vi "_FPGA Auxiliary Update.vi"(5 "Setting Value":sgl, 6 "Command Type":i32) -> (0 "error out":errorcluster, 1 "Return Value":string)   [LabVIEW 2015]
uses:
  Type/_Syringe Pump Command.ctl
  Type/_Pump Parameter.ctl
  _RT Global.vi
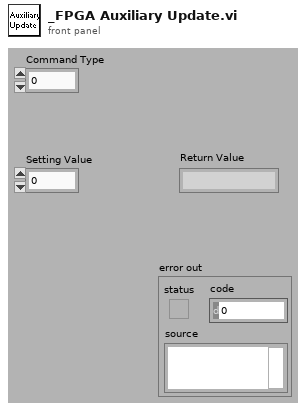
[diagram p1: front panel]
types:
  T1 = typedef "_Syringe Pump Command.ctl" = enum16{"start", "stop", "pause", "restart", "help", "set units", "set diameter", "set rate", "set time", "set volume", "set delay", "save setting", "read limit parameter", "view parameter", "status"}
  T2 = typedef "_Pump Parameter.ctl" = enum16{"Turn Pump Motor On", "Turn Pump Motor Off", "Read Pump Oil Deficiency", "Read Rotation Switch Point Attained", "Read Ele. Drive Over Temperature", "Read Pump Over Temperature", "Read Set Rotation Speed Attained", "Read Turbopump Accelerates", "Read Actual Rotation Speed in Hz", "Read Motor Current in A", "Read Operating Hours in h", "Read Motor Voltage in V", "Read Motor Power in W", "Set Rotation Speed Switchpoint in %", "Clear Error", "Read Error Code", "Read Bearing Temperature", "Read Hardware Version", "Read Firmware Version", "Read Operating Hours (Drive)", "Read Rotational Speed (rpm)", "Read Power Stage Temperature", "Read Electronics Temperature", "Read Upper Pump Temperature", "Read Motor Temperature", "Read Error Code History, 1", "Read Error Code History, 2", "Read Error Code History, 3", "Read Error Code History, 4", "Read Error Code History, 5", "Read Error Code History, 6", "Read Error Code History, 7", "Read Error Code History, 8", "Read Error Code History, 9", "Read Error Code History, 10"}
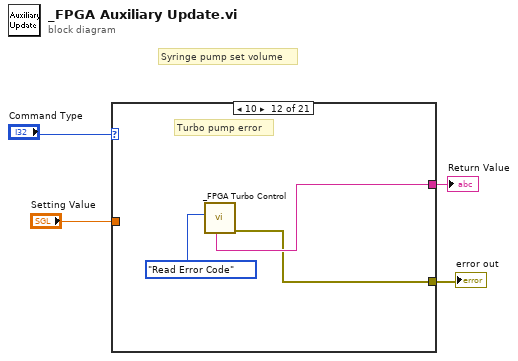
[diagram p0: block diagram]
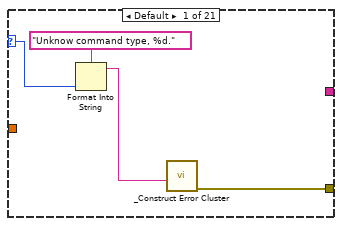
[diagram p2: hidden frame]
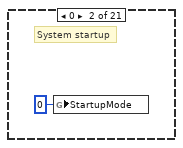
[diagram p3: hidden frame]
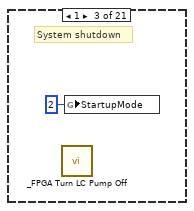
[diagram p4: hidden frame]
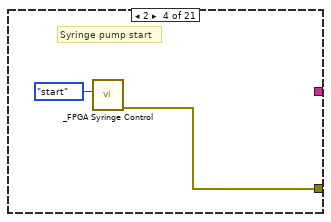
[diagram p5: hidden frame]
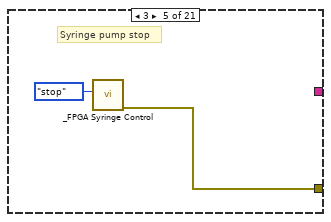
[diagram p6: hidden frame]
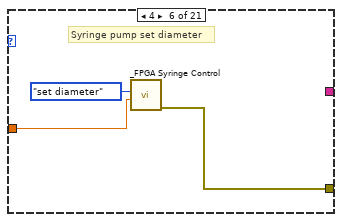
[diagram p7: hidden frame]
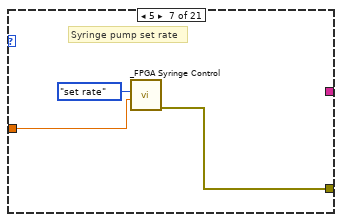
[diagram p8: hidden frame]
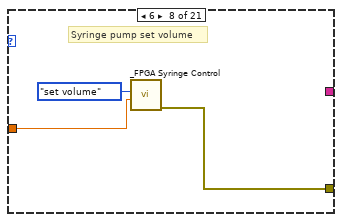
[diagram p9: hidden frame]
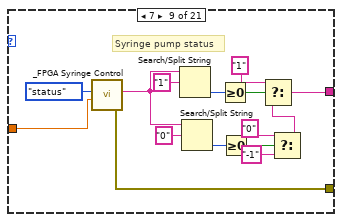
[diagram p10: hidden frame]
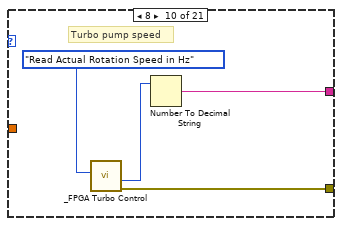
[diagram p11: hidden frame]
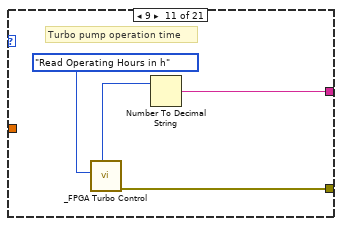
[diagram p12: hidden frame]
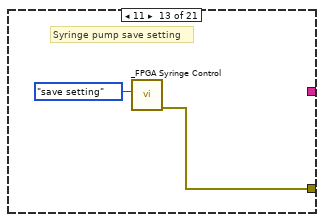
[diagram p13: hidden frame]
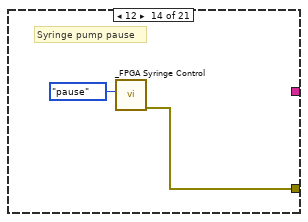
[diagram p14: hidden frame]
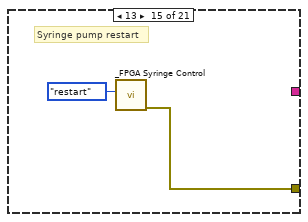
[diagram p15: hidden frame]
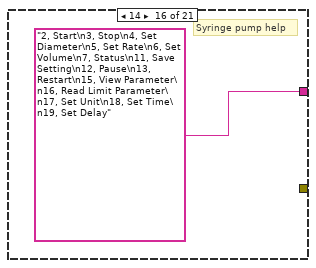
[diagram p16: hidden frame]
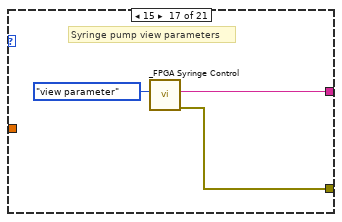
[diagram p17: hidden frame]
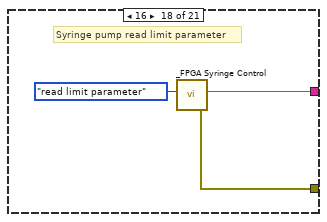
[diagram p18: hidden frame]
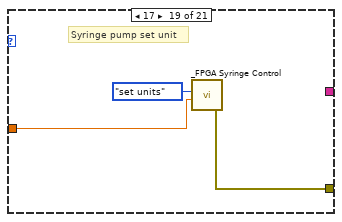
[diagram p19: hidden frame]
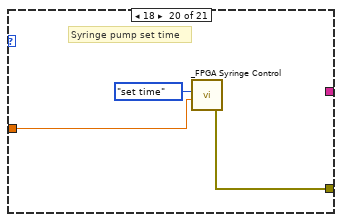
[diagram p20: hidden frame]
diagram:
  # "Syringe pump set volume"
  n1 = case shown="10" "Command Type" {
    selector: "Command Type" -> [w8 _ _ _ _ _ _ _ _ _ _ _ _ _ _ _ _ _ _ _ _]
    tunnel: [w5 _ _ w12 w14 w17 w20 w23 w38 w41 w45 w47 w51 w53 w55 _ w59 w62 w65 w68 w71] -> w2
    tunnel: "Setting Value" -> [_ _ _ _ _ w15 w18 w21 w36 _ _ _ _ _ _ _ _ _ w63 w66 w69]
    tunnel: [_ _ _ _ _ _ _ _ w25 w39 w44 w48 _ _ _ "2, Start\n3, Stop\n4, Set Diameter\n5, Set Rate\n6, Set Volume\n7, Status\n11, Save Setting\n12, Pause\n13, Restart\n15, View Parameter\n16, Read Limit Parameter\n17, Set Unit\n18, Set Time\n19, Set Delay" ("Reply") w57 w60 _ _ _] -> w1
    frame Default {
      n2 = Format Into String(format string="Unknow command type, %d.", w8) -> (resulting string=w6:string)  [unwired: 2 in, 1 out]
      n3 = call "_Construct Error Cluster.vi"("reason"=w6) -> ("error out"=w5:errorcluster)  [unwired: 3 in, 3 out]
    }
    frame 0 {
      # "System startup"
      n4 = global write "_RT Global.vi" "StartupMode"(u8 0 ("StartupMode")) -> ()
    }
    frame 1 {
      # "System shutdown"
      n5 = call "_FPGA Turn LC Pump Off.vi"() -> ()  [unwired: 2 in]
      n6 = global write "_RT Global.vi" "StartupMode"(u8 2 ("StartupMode")) -> ()
    }
    frame 2 {
      # "Syringe pump start"
      n7 = call "_FPGA Syringe Control.vi"("Pump Command"=_Syringe_Pump_Command."start") -> ("error out"=w12:errorcluster)  [unwired: 5 in, 2 out]
    }
    frame 3 {
      # "Syringe pump stop"
      n8 = call "_FPGA Syringe Control.vi"("Pump Command"=_Syringe_Pump_Command."stop") -> ("error out"=w14:errorcluster)  [unwired: 5 in, 2 out]
    }
    frame 4 {
      # "Syringe pump set diameter"
      n9 = call "_FPGA Syringe Control.vi"("Input Value"=w15, "Pump Command"=_Syringe_Pump_Command."set diameter") -> ("error out"=w17:errorcluster)  [unwired: 4 in, 2 out]
    }
    frame 5 {
      # "Syringe pump set rate"
      n10 = call "_FPGA Syringe Control.vi"("Input Value"=w18, "Pump Command"=_Syringe_Pump_Command."set rate") -> ("error out"=w20:errorcluster)  [unwired: 4 in, 2 out]
    }
    frame 6 {
      # "Syringe pump set volume"
      n11 = call "_FPGA Syringe Control.vi"("Input Value"=w21, "Pump Command"=_Syringe_Pump_Command."set volume") -> ("error out"=w23:errorcluster)  [unwired: 4 in, 2 out]
    }
    frame 7 {
      # "Syringe pump status"
      n12 = call "_FPGA Syringe Control.vi"("Input Value"=w36, "Pump Command"=_Syringe_Pump_Command."status") -> ("error out"=w38:errorcluster, "Reply"=w26:string)  [unwired: 4 in, 1 out]
      n13 = Search/Split String(string=w26, search string/char (-)="1") -> (offset of match=w33:i32)  [unwired: 3 out]
      n14 = Search/Split String(string=w26, search string/char (-)="0") -> (offset of match=w32:i32)  [unwired: 3 out]
      n15 = Greater Or Equal To 0?(x=w33) -> (x >= 0?=w31:bool)
      n16 = Greater Or Equal To 0?(x=w32) -> (x >= 0?=w29:bool)
      n17 = Select(t="0" ("search string/char (-)"), s=w29, f="-1") -> (s? t:f=w24:string)
      n18 = Select(t="1" ("search string/char (-)"), s=w31, f=w24) -> (s? t:f=w25:string)
    }
    frame 8 {
      # "Turbo pump speed"
      n19 = call "_FPGA Turbo Control.vi"("Command"=_Pump_Parameter."Read Actual Rotation Speed in Hz") -> ("error out"=w41:errorcluster, "Speed"=w40:i32)  [unwired: 3 in, 4 out]
      n20 = Number To Decimal String(number=w40) -> (decimal integer string=w39:string)  [unwired: 1 out]
    }
    frame 9 {
      # "Turbo pump operation time"
      n21 = call "_FPGA Turbo Control.vi"("Command"=_Pump_Parameter."Read Operating Hours in h") -> ("error out"=w45:errorcluster, "Time"=w43:i32)  [unwired: 3 in, 4 out]
      n22 = Number To Decimal String(number=w43) -> (decimal integer string=w44:string)  [unwired: 1 out]
    }
    frame 10 {
      # "Turbo pump error"
      n23 = call "_FPGA Turbo Control.vi"("Command"=_Pump_Parameter."Read Error Code") -> ("error out"=w47:errorcluster, "Error Code"=w48:string)  [unwired: 3 in, 4 out]
    }
    frame 11 {
      # "Syringe pump save setting"
      n24 = call "_FPGA Syringe Control.vi"("Pump Command"=_Syringe_Pump_Command."save setting") -> ("error out"=w51:errorcluster)  [unwired: 5 in, 2 out]
    }
    frame 12 {
      # "Syringe pump pause"
      n25 = call "_FPGA Syringe Control.vi"("Pump Command"=_Syringe_Pump_Command."pause") -> ("error out"=w53:errorcluster)  [unwired: 5 in, 2 out]
    }
    frame 13 {
      # "Syringe pump restart"
      n26 = call "_FPGA Syringe Control.vi"("Pump Command"=_Syringe_Pump_Command."restart") -> ("error out"=w55:errorcluster)  [unwired: 5 in, 2 out]
    }
    frame 14 {
      # "Syringe pump help"
    }
    frame 15 {
      # "Syringe pump view parameters"
      n27 = call "_FPGA Syringe Control.vi"("Pump Command"=_Syringe_Pump_Command."view parameter") -> ("error out"=w59:errorcluster, "Reply"=w57:string)  [unwired: 5 in, 1 out]
    }
    frame 16 {
      # "Syringe pump read limit parameter"
      n28 = call "_FPGA Syringe Control.vi"("Pump Command"=_Syringe_Pump_Command."read limit parameter") -> ("error out"=w62:errorcluster, "Reply"=w60:string)  [unwired: 5 in, 1 out]
    }
    frame 17 {
      # "Syringe pump set unit"
      n29 = call "_FPGA Syringe Control.vi"("Input Value"=w63, "Pump Command"=_Syringe_Pump_Command."set units") -> ("error out"=w65:errorcluster)  [unwired: 4 in, 2 out]
    }
    frame 18 {
      # "Syringe pump set time"
      n30 = call "_FPGA Syringe Control.vi"("Input Value"=w66, "Pump Command"=_Syringe_Pump_Command."set time") -> ("error out"=w68:errorcluster)  [unwired: 4 in, 2 out]
    }
    frame 19 {
      # "Syringe pump set time"
      n31 = call "_FPGA Syringe Control.vi"("Input Value"=w69, "Pump Command"=_Syringe_Pump_Command."set delay") -> ("error out"=w71:errorcluster)  [unwired: 4 in, 2 out]
    }
  }
  "error out" <- w2
  "Return Value" <- w1
